vi "Requests.vi"(8 "error in (no error)":errorcluster, 9 "write enable":bool=TRUE, 11 "TEST in":refnum<class "TEST.lvclass">) -> (0 "error out":errorcluster, 3 "TEST out":refnum<class "TEST.lvclass">)   [LabVIEW 2021, in "TEST.lvclass"]
uses:
  TEST.lvclass
  D:/my_projects/projects/Algorithms/Labview/21/Modbus/MB_TCP2/MB_TCP.lvclass
  NI_modbus_upd/TCP/tcp timeouts.ctl
  MB_TCP.lvclass/MB_TCP.ctl
  NI_modbus_upd/TCP/TCP.lvclass/TCP.ctl
  NI_modbus_upd/TCP/TCP.lvclass
  MB_TCP.lvclass
  ICPCON Registers/ICPCON Registers.lvlib
panel:
  out "timeouts":T1={"connect timeout"=60000, "write timeout"=10000, "read timeout"=10000}
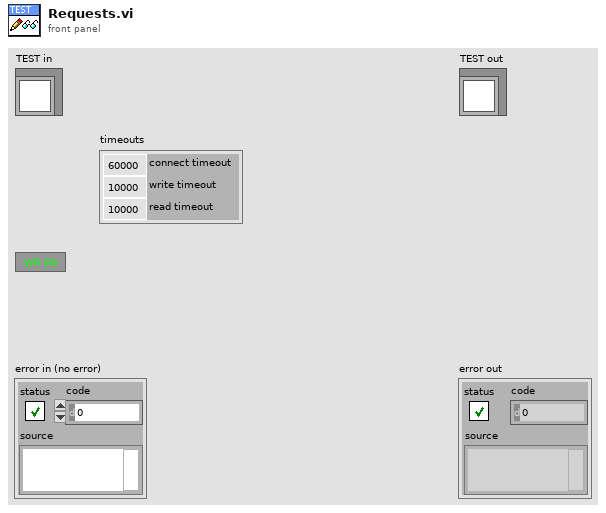
[diagram p1: front panel]
types:
  T1 = typedef "TCP.lvclass/tcp timeouts.ctl" = cluster{"connect timeout":i32, "write timeout":i32, "read timeout":i32}
  T2 = typedef "ICPCON Registers.lvlib/ICPCON Data.ctl" = cluster{"UTF":refnum<data-value>, "DI":refnum<data-value>, "DW":refnum<data-value>, "DO":refnum<data-value>, "IR":refnum<data-value>, "WR":refnum<data-value>, "OR":refnum<data-value>, "modified":refnum<data-value>}
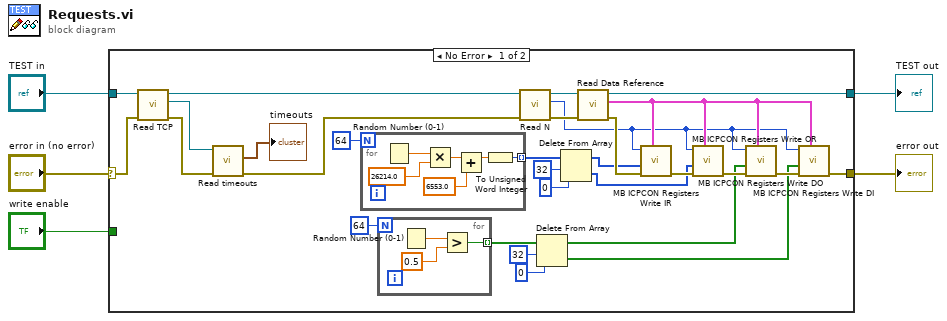
[diagram p0: block diagram]
diagram:
  n1 = case shown="No Error" "error in (no error)" {
    selector: "error in (no error)" -> [w29 w45]
    tunnel: [w31 w45] -> w1
    tunnel: [w27 w44] -> w4
    tunnel: "TEST in" -> [w30 w44]
    tunnel: "write enable" -> [_ _]
    frame No Error {
      n2 = call "Read TCP.vi"("error in (no error)"=w29, "MB_TCP in"=w30) -> ("error out"=w24:errorcluster, "TCP"=w25:refnum<class "TCP.lvclass">, "MB_TCP out"=w28:refnum<class "TEST.lvclass">)  [unwired: 7 in]
      n3 = call "Read timeouts.vi"("error in (no error)"=w24, "TCP in"=w25) -> ("error out"=w22:errorcluster, "timeouts"=→"timeouts":T1)  [unwired: 7 in, 1 out]
      n4 = for {
        N: 64 -> [_]
        tunnel: [w37] -> w17 mode=indexing
        n5 = Random Number (0-1)() -> (number: 0 to 1=w40:dbl)
        n6 = Multiply(x=w40, y=26214.0) -> (x*y=w38:dbl)
        n7 = Add(x=w38, y=6553.0) -> (x+y=w36:dbl)
        n8 = To Unsigned Word Integer(number=w36) -> (unsigned 16bit integer=w37:u16)
      }
      n9 = for {
        N: 64 -> [_]
        tunnel: [w41] -> w16 mode=indexing
        n10 = Random Number (0-1)() -> (number: 0 to 1=w43:dbl)
        n11 = Greater?(x=w43, y=0.5) -> (0:w41:bool)
      }
      n12 = call "Read N.vi"("error in (no error)"=w22, "MB_TCP in"=w28) -> ("error out"=w34:errorcluster, "N"=w18:i32, "MB_TCP out"=w33:refnum<class "TEST.lvclass">)  [unwired: 7 in]
      n13 = Delete From Array(array=w16, length=32, index=0) -> (deleted portion=w6:bool[], array with subset deleted=w7:bool[])
      n14 = Delete From Array(array=w17, length=32, index=0) -> (deleted portion=w8:u16[], array with subset deleted=w9:u16[])
      n15 = call "Read Data Reference.vi"("error in (no error)"=w34, "MB_TCP in"=w33) -> ("error out"=w26:errorcluster, "Data"=w21:T2, "MB_TCP out"=w27:refnum<class "TEST.lvclass">)  [unwired: 7 in]
      n16 = call "MB ICPCON Registers Write IR.vi"("Data Reference"=w21, "error in (no error)"=w26, "Words In"=w9, "N"=w18) -> ("error out"=w20:errorcluster)  [unwired: 7 in]
      n17 = call "MB ICPCON Registers Write OR.vi"("Data Reference"=w21, "error in (no error)"=w20, "Words In"=w8, "N"=w18) -> ("error out"=w19:errorcluster)  [unwired: 7 in]
      n18 = call "MB ICPCON Registers Write DO.vi"("Data Reference"=w21, "error in (no error)"=w19, "Bits In"=w7, "N"=w18) -> ("error out"=w32:errorcluster)  [unwired: 7 in]
      n19 = call "MB ICPCON Registers Write DI.vi"("Data Reference"=w21, "error in (no error)"=w32, "Bits In"=w6, "N"=w18) -> ("error out"=w31:errorcluster)  [unwired: 7 in]
    }
    frame Error {
    }
  }
  "error out" <- w1
  "TEST out" <- w4
